vi "WaveFormGenerator.vi"(0 "Enable":bool, 1 "Ref Chan Delay (s)":dbl, 5 "Samples Per Channel":dbl, 7 "Min End of Wave Off samples":dbl, 9 "Clock Rate (Hz)":dbl, 11 "Trigger Width (s)":dbl, 13 "Relative Chan Delay (s)":dbl) -> (4 "OutArray":bool[][](array[boolean]))   [LabVIEW 2016]
panel:
  # "This will ensure that the waveform is held to zero \nfor this many samples before end of wave"
  # "Signal Boolean Array"
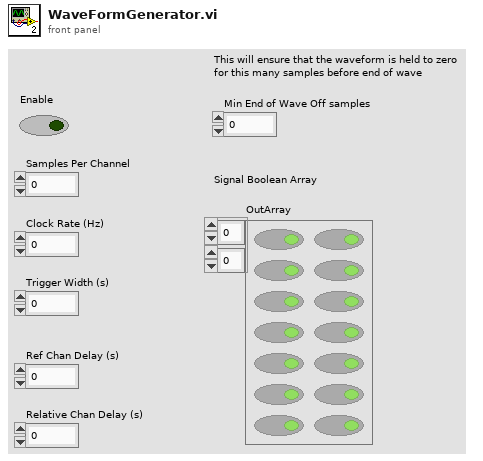
[diagram p1: front panel]
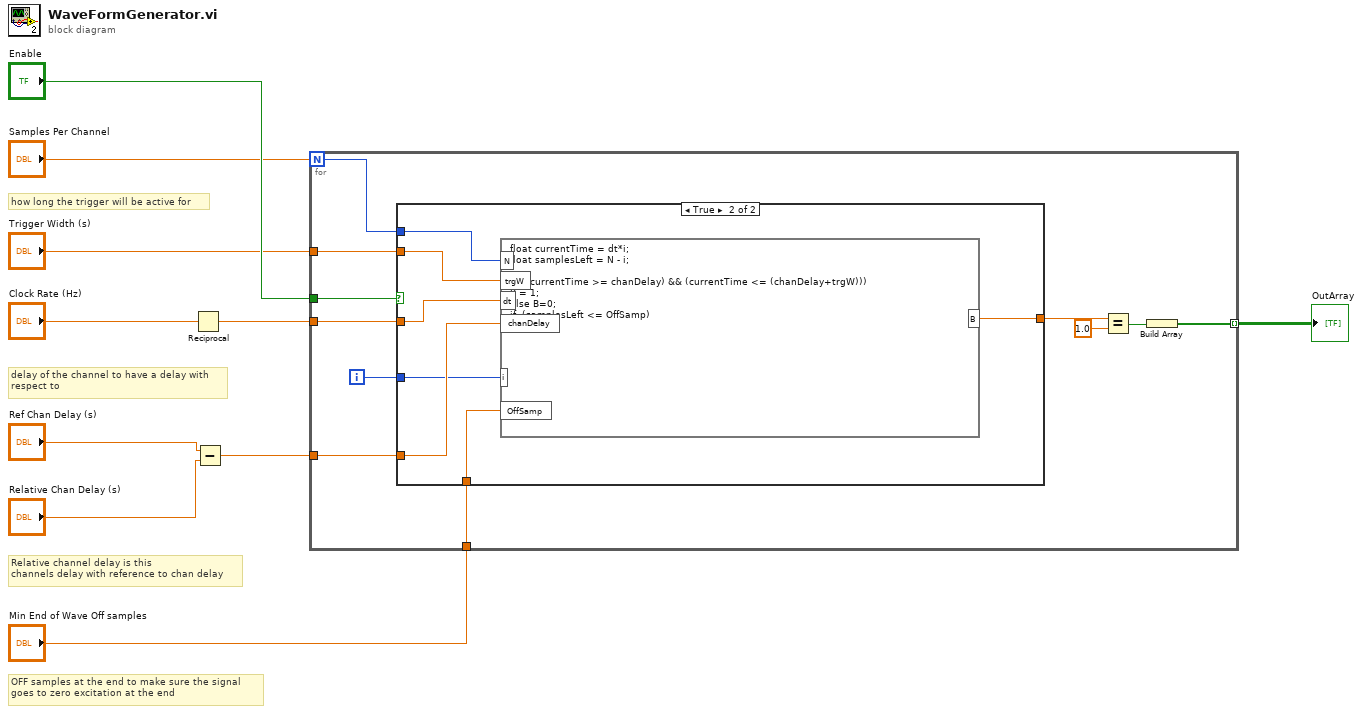
[diagram p0: block diagram]
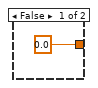
[diagram p2: hidden frame]
diagram:
  # "OFF samples at the end to make sure the signal \ngoes to zero excitation at the end"
  # "how long the trigger will be active for"
  # "Relative channel delay is this \nchannels delay with reference to chan delay"
  # "delay of the channel to have a delay with\nrespect to"
  n1 = Reciprocal(x="Clock Rate (Hz)") -> (1/x=w4:dbl)
  n2 = Subtract(x="Ref Chan Delay (s)", y="Relative Chan Delay (s)") -> (x-y=w5:dbl)
  n3 = for {
    N: "Samples Per Channel" -> [w11]
    tunnel: "Enable" -> [w21]
    tunnel: w5 -> [w20]
    tunnel: w4 -> [w19]
    tunnel: "Trigger Width (s)" -> [w18]
    tunnel: "Min End of Wave Off samples" -> [w16]
    tunnel: [w12] -> w1 mode=indexing
    i -> [w17]
    n4 = case shown="True" w21 {
      tunnel: w20 -> [_ w29]
      tunnel: w19 -> [_ w28]
      tunnel: w18 -> [_ w27]
      tunnel: w17 -> [_ w26]
      tunnel: w16 -> [_ w25]
      tunnel: [0.0 ("B") w24] -> w15
      tunnel: w11 -> [_ w23]
      frame False {
      }
      frame True {
        n5 = formula code="float currentTime = dt*i;\nfloat samplesLeft = N - i;\n\nif ( (currentTime >= chanDelay) && (currentTime <= (chanDelay+trgW)))\nB = 1;\nelse B=0;\nif  (samplesLeft <= OffSamp)\nB = 0;"("dt"=w28, "chanDelay"=w29, "trgW"=w27, "i"=w26, "OffSamp"=w25, "N"=w23) -> ("B"=w24:dbl)
      }
    }
    n6 = Equal?(x=w15, y=1.0) -> (x = y?=w14:bool)
    n7 = Build Array(w14) -> (w12:bool[])
  }
  "OutArray" <- w1
